vi "Subpanel - Helper.vi"() -> ()   [LabVIEW 2016]
uses:
  <vilib>/Utility/error.llb/DialogType.ctl
  <vilib>/SLL Toolkit/SLL Queued State Machine/Queue Driver/Create Queue.vi
  <vilib>/SLL Toolkit/SLL Queued State Machine/Queue Driver/Enqueue an Item to Queue.vi
  <vilib>/SLL Toolkit/SLL Queued State Machine/Queue Driver/Dequeue Queue.vi
  <vilib>/SLL Toolkit/SLL Queued State Machine/Queue Driver/Enqueue N Items.vi
  <vilib>/SLL Toolkit/SLL Queued State Machine/Queue Driver/Flush Queue.vi
  <vilib>/SLL Toolkit/SLL Queued State Machine/Queue Driver/Release Queue.vi
  <vilib>/SLL Toolkit/SLL Queued State Machine/SLL QSM.lvlib
panel:
  in  "STOP":bool
  in  "VI to load":string(combo)="Latch boolean simulation"
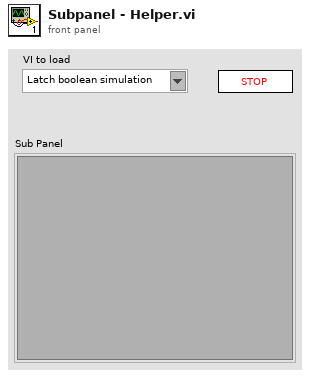
[diagram p1: front panel]
types:
  T1 = cluster{"Flags":cluster{"Source Code?":bool, "VI Inserted?":bool}, "VI Details":string[][], "VI Ref":refnum<vi>}
  T2 = typedef "DialogType.ctl" = u16
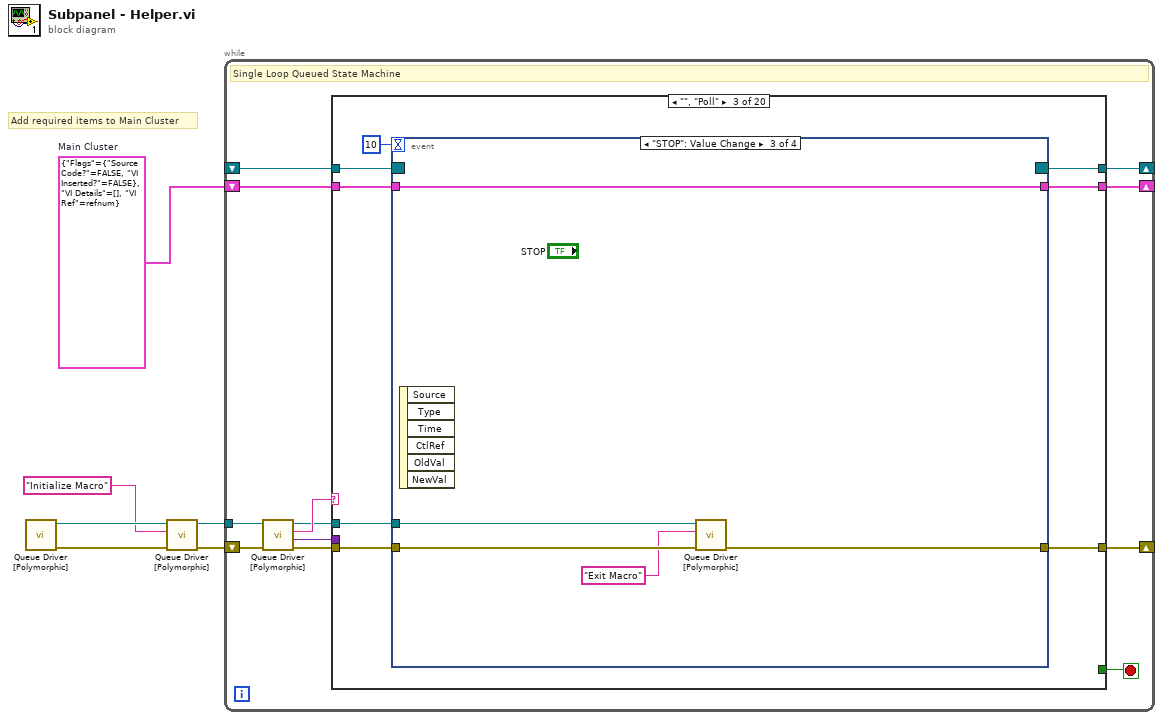
[diagram p0: block diagram]
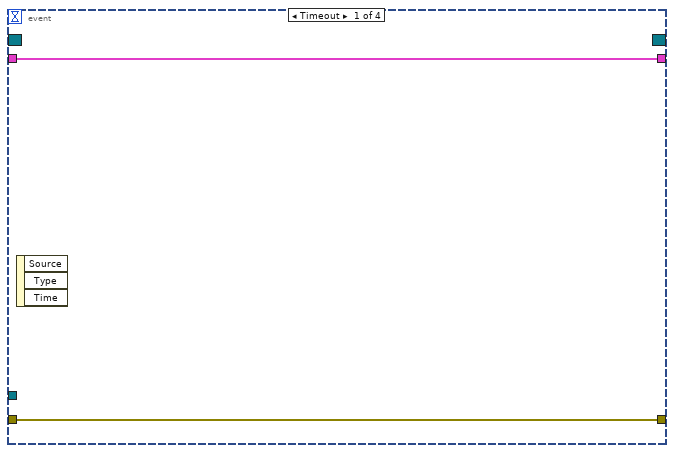
[diagram p4: hidden frame]
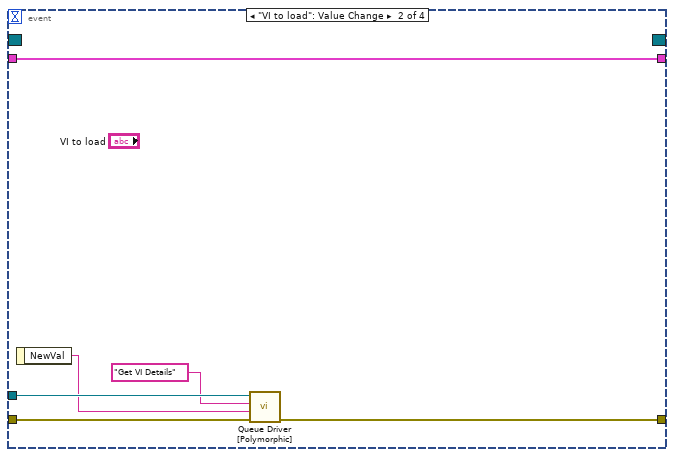
[diagram p5: hidden frame]
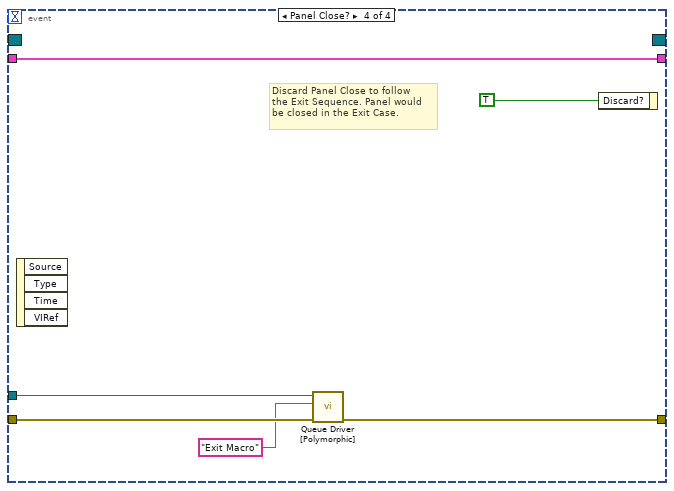
[diagram p6: hidden frame]
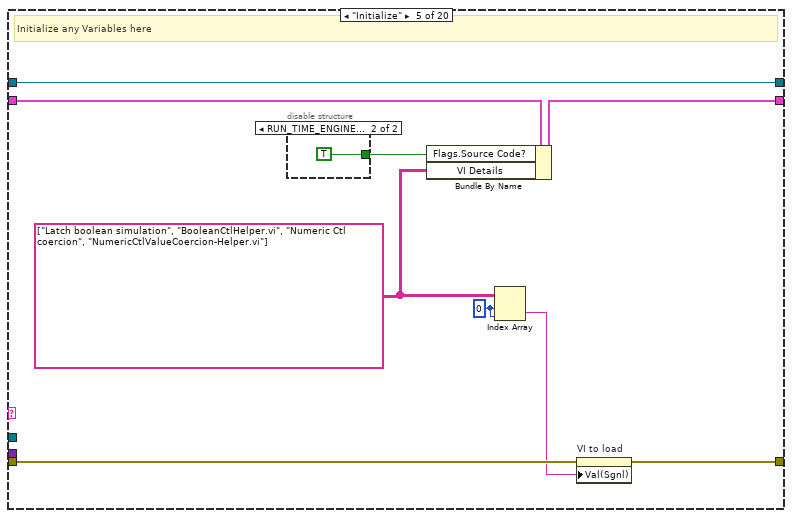
[diagram p8: hidden frame]
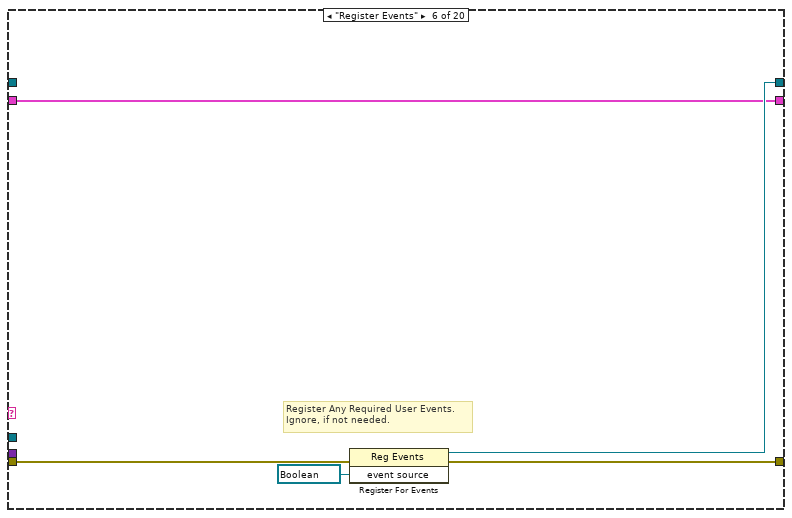
[diagram p10: hidden frame]
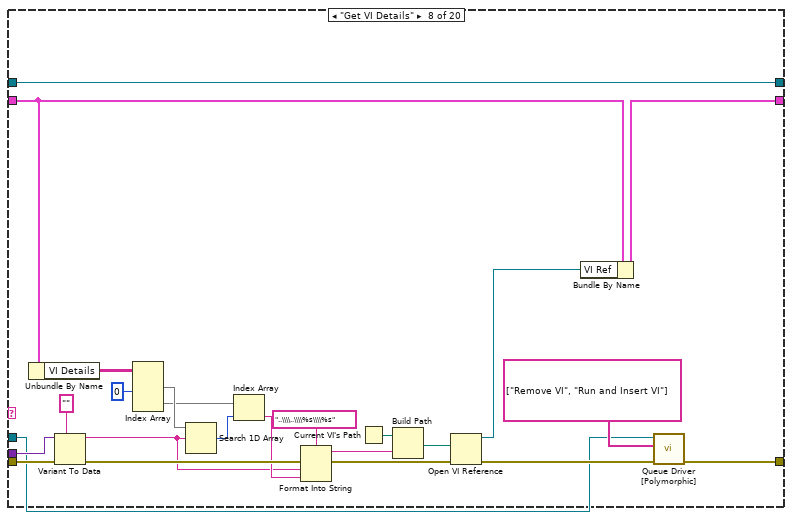
[diagram p12: hidden frame]
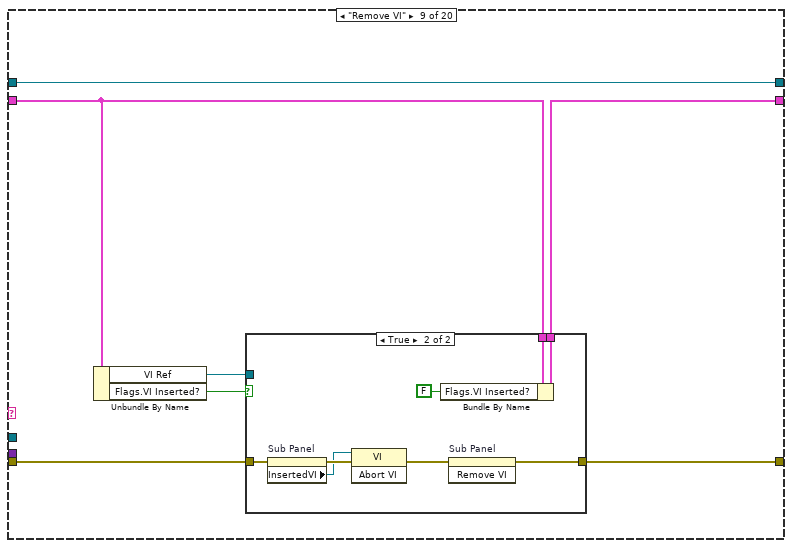
[diagram p13: hidden frame]
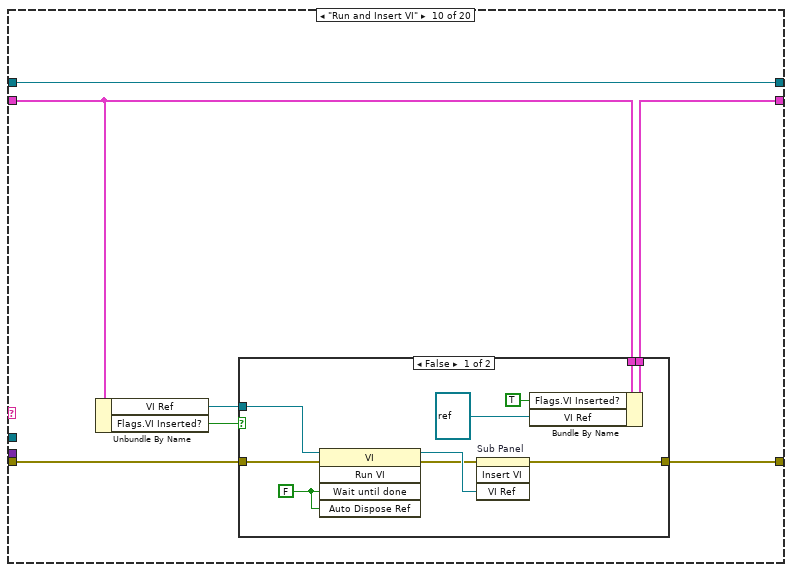
[diagram p15: hidden frame]
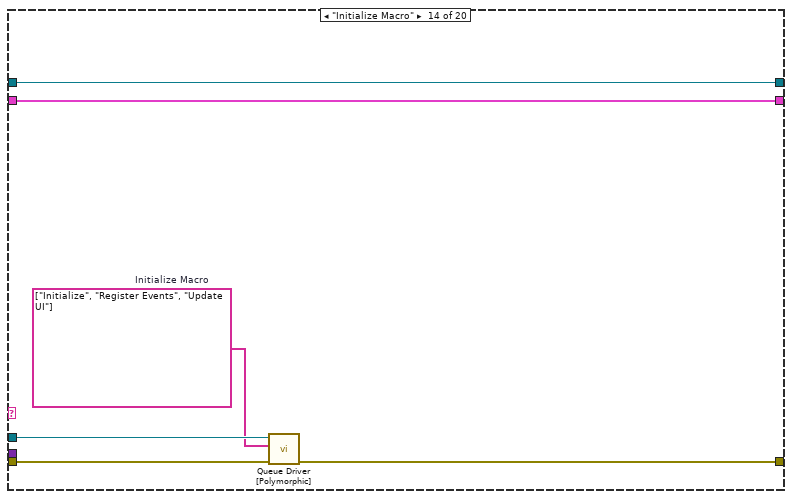
[diagram p20: hidden frame]
diagram:
  w3 = T1 {"Flags"={"Source Code?"=FALSE, "VI Inserted?"=FALSE}, "VI Details"=[], "VI Ref"=refnum}  # Main Cluster
  # "Add required items to Main Cluster"
  n1 = call-poly <vilib>:"Queue Driver [Polymorphic].vi"() -> ("Error Out"=w1:errorcluster, "Queue Ref"=w5:refnum<queue>)  [unwired: 10 in]
  n2 = call-poly <vilib>:"Queue Driver [Polymorphic].vi"("Error In"=w1, "Item to Add"="Initialize Macro", "Queue Ref In"=w5) -> ("Error Out"=w2:errorcluster, "Queue Ref Out"=w6:refnum<queue>)  [unwired: 7 in]
  n3 = while "SLL Queued State Machine" {
    shift-right: [w16] -> _
    shift-left: w2 -> [w18]
    shift-right: [w14] -> _
    shift-left: _ -> [w13]
    shift-right: [w12] -> _
    shift-left: w3 -> [w11]
    tunnel: w6 -> [w9]
    stop <- w15 stop-if-true
    # "Single Loop Queued State Machine"
    n4 = call-poly <vilib>:"Queue Driver [Polymorphic].vi"("Error In"=w18, "Queue Ref In"=w9) -> ("Error Out"=w17:errorcluster, "Data"=w7:variant, "Dequeue"=w10:string, "Queue Ref Out"=w8:refnum<queue>)  [unwired: 6 in]
    n5 = case "QSM Case Structure" shown="\"\", \"Poll\"" w10 {
      selector: w10 -> [_ _ _ _ _ _ _ _ _ _ _ _ _ _ _ _ w157 _ _ _]
      tunnel: w17 -> [w21 w24 w30 w54 w58 w69 w72 w96 w102 w120 w135 w138 w141 w145 w151 w156 w160 w172 w175 w188]
      tunnel: [w21 w24 w31 w54 w59 w68 w72 w77 w101 w117 w135 w138 w141 w144 w150 w156 w163 w170 w175 w184] -> w16
      tunnel: [_ _ _ _ _ _ _ _ _ _ _ _ _ _ _ _ _ _ _ TRUE] -> w15
      tunnel: [w20 w23 w29 w53 w63 w67 w71 w95 w103 w119 w134 w137 w140 w147 w153 w155 w166 w169 w174 w187] -> w14
      tunnel: w13 -> [w20 w23 w28 w53 w63 _ w71 w95 w103 w119 w134 w137 w140 w147 w153 w155 w166 w169 w174 w187]
      tunnel: [w19 w22 w26 w52 w60 w66 w70 w75 w97 w115 w133 w136 w139 w146 w152 w154 w165 w168 w173 w186] -> w12
      tunnel: w11 -> [w19 w22 w27 w52 w61 w66 w70 w76 w98 w116 w133 w136 w139 w146 w152 w154 w165 w168 w173 w186]
      tunnel: w8 -> [_ _ w25 _ _ _ _ w73 _ _ _ _ _ w143 w148 _ _ _ _ w177]
      tunnel: w7 -> [_ _ _ _ _ _ _ w93 _ _ _ _ _ _ _ _ _ _ _ _]
      frame "/--------------- Read Me -----------------/" {
        # "General Purpose Queue Based State Machine for Any Use Case (main application, module, pop up message etc)\n\nAdvantages:\n1. Lean Project Code Base (dependencies are in vilib).\n2. This template can be safely used in multiple parallel running modules without any issues.\n3. This template can also be safely used even in cases where the VI is configured to be a clone, where multiple \ninstances of the VI could be executing concurrently.\n\nHow to Use:\n1. Add necessary items to the Main Cluster.\n2. Use the Polymorphic Queue Driver for doing any queue operations. \n3. Add any required user events in the \"Register Events\" case. Ignore if not needed.\n4. Use \"Macros\" section for defining any list of state calls, which could be used in multiple places. \nEx: Initialize Macro, might be needed if we need to any reinitialization."
      }
      frame "/------------------ Poll -------------------/" {
      }
      frame "", "Poll" {
        n6 = event shown="[2] \"STOP\": Value Change" {
          selector: w28 -> [_ _ _ _]
          dyn-events: [_ _ _ _] -> w29
          timeout: 10 -> [_ _ _ _]
          tunnel: [w34 w37 w44 w50] -> w31
          tunnel: w30 -> [w34 w38 w45 w51]
          tunnel: w27 -> [w33 w40 w43 w49]
          tunnel: [w33 w40 w43 w49] -> w26
          tunnel: w25 -> [_ w39 w42 w47]
          event Timeout {
            n7 = event-data() -> ()  [unwired: 1 in, 3 out]
          }
          event "VI to load": Value Change {
            n8 = event-data() -> ("NewVal"=w35:string)  [unwired: 1 in]
            n9 = call-poly <vilib>:"Queue Driver [Polymorphic].vi"("Error In"=w38, "Data (Optional)"=w35, "Item to Add"="Get VI Details", "Queue Ref In"=w39) -> ("Error Out"=w37:errorcluster)  [unwired: 6 in, 1 out]
          }
          event "STOP": Value Change {
            n10 = event-data() -> ()  [unwired: 1 in, 6 out]
            n11 = call-poly <vilib>:"Queue Driver [Polymorphic].vi"("Error In"=w45, "Item to Add"="Exit Macro" ("Enqueue"), "Queue Ref In"=w42) -> ("Error Out"=w44:errorcluster)  [unwired: 7 in, 1 out]
          }
          event Panel Close? {
            # "Discard Panel Close to follow\nthe Exit Sequence. Panel would\nbe closed in the Exit Case."
            n12 = event-data() -> ()  [unwired: 1 in, 4 out]
            n13 = call-poly <vilib>:"Queue Driver [Polymorphic].vi"("Error In"=w51, "Item to Add"="Exit Macro" ("Enqueue"), "Queue Ref In"=w47) -> ("Error Out"=w50:errorcluster)  [unwired: 7 in, 1 out]
            n14 = event-data("Discard?"=TRUE) -> ()  [unwired: 1 in, 1 out]
          }
        }
      }
      frame "/--------------- Initialize -----------------/" {
      }
      frame "Initialize" {
        w56 = 0 ("index (row)")
        w57 = string[][] [["Latch boolean simulation", "BooleanCtlHelper.vi"], ["Numeric Ctl coercion", "NumericCtlValueCoercion-Helper.vi"]]
        # "Initialize any Variables here"
        n15 = disable-structure shown="RUN_TIME_ENGINE==False" {
          disable-tunnel: [_ TRUE] -> w62
          frame condition #0 {
          }
          frame condition #1 (active) {
          }
        }
        n16 = Bundle By Name(cluster=w61, "Flags.Source Code?"=w62, "VI Details"=w57) -> (w60:T1)
        n17 = Index Array(array=w57, index (row)=w56, index (col)=w56) -> (element=w55:string)
        n18 = property on="VI to load" class="CmbBox"(error in=w58, "Val(Sgnl)"=w55) -> (error out=w59:errorcluster)  [unwired: 1 in, 1 out]
      }
      frame "Register Events" {
        # "Register Any Required User Events. \nIgnore, if not needed."
        n19 = register-events(error in=w69, refnum<vi> refnum ("event source")) -> (reference out=w67:refnum<event-registration>, error out=w68:errorcluster)  [unwired: 1 in]
      }
      frame "/---------- Custom Case Splitter ----------/" {
      }
      frame "Get VI Details" {
        n20 = Unbundle By Name(w76) -> ("VI Details"=w91:string[][])
        n21 = Variant To Data(error in=w96, type="", Variant=w93) -> (data=w81:string, error out=w85:errorcluster)
        n22 = Index Array(array=w91, index (col) #1=0 ("disabled index (col)")) -> (element #1=w89:string[], element #2=w88:string[])  [unwired: 3 in]
        n23 = Search 1D Array(1D array=w89, element=w81) -> (index of element=w87:i32)  [unwired: 1 in]
        n24 = Index Array(array=w88, index=w87) -> (element=w83:string)
        n25 = Format Into String(format string="..\\\\..\\\\%s\\\\%s", error in=w85, w81, w83) -> (resulting string=w80:string, error out=w84:errorcluster)  [unwired: 1 in]
        n26 = Current VI's Path() -> (path=w86:path)
        n27 = Build Path(base path=w86, name or relative path=w80) -> (appended path=w79:path)
        n28 = Open VI Reference(vi path=w79, error in (no error)=w84) -> (vi reference=w74:refnum<vi>, error out=w78:errorcluster)  [unwired: 4 in]
        n29 = Bundle By Name(cluster=w76, "VI Ref"=w74) -> (w75:T1)
        n30 = call-poly <vilib>:"Queue Driver [Polymorphic].vi"("Error In"=w78, "Enqueue N"=string[] ["Remove VI", "Run and Insert VI"], "Queue Ref In"=w73) -> ("Error Out"=w77:errorcluster)  [unwired: 7 in, 1 out]
      }
      frame "Remove VI" {
        n31 = Unbundle By Name(w98) -> ("VI Ref"=w99:refnum<vi>, "Flags.VI Inserted?"=w100:bool)
        n32 = case shown="True" w100 {
          tunnel: w102 -> [w105 w113]
          tunnel: [w105 w109] -> w101
          tunnel: w99 -> [_ _]
          tunnel: w98 -> [w104 w108]
          tunnel: [w104 w107] -> w97
          frame False {
          }
          frame True {
            n33 = property on="Sub Panel" class="SubPnl"(error in=w113) -> (error out=w112:errorcluster, "InsertedVI"=w111:refnum<vi>)  [unwired: 1 in, 1 out]
            n34 = invoke class="VI" method="Abort VI"(reference=w111, error in=w112) -> (error out=w110:errorcluster)  [unwired: 1 in, 2 out]
            n35 = Bundle By Name(cluster=w108, "Flags.VI Inserted?"=FALSE) -> (w107:T1)
            n36 = invoke on="Sub Panel" class="SubPnl" method="Remove VI"(error in=w110) -> (error out=w109:errorcluster)  [unwired: 2 in, 2 out]
          }
        }
      }
      frame "Run and Insert VI" {
        n37 = Unbundle By Name(w116) -> ("VI Ref"=w118:refnum<vi>, "Flags.VI Inserted?"=w114:bool)
        n38 = case shown="False" w114 {
          tunnel: w120 -> [w130 w131]
          tunnel: w118 -> [w129 _]
          tunnel: [w126 w131] -> w117
          tunnel: w116 -> [w123 w132]
          tunnel: [w122 w132] -> w115
          frame False {
            w125 = FALSE ("Wait Until Done")
            n39 = invoke class="VI" method="Run VI"(reference=w129, error in=w130, "Wait until done"=w125, "Auto Dispose Ref"=w125) -> (reference out=w128:refnum<vi>, error out=w127:errorcluster)  [unwired: 1 in, 3 out]
            n40 = invoke on="Sub Panel" class="SubPnl" method="Insert VI"(error in=w127, "VI Ref"=w128) -> (error out=w126:errorcluster)  [unwired: 2 in, 3 out]
            n41 = Bundle By Name(cluster=w123, "Flags.VI Inserted?"=TRUE, "VI Ref"=refnum<vi> refnum) -> (w122:T1)
          }
          frame True {
          }
        }
      }
      frame "/-------------- User Interface --------------/" {
        # "Duplicate this case to create additional case splitters for readability"
      }
      frame "Update UI" {
        # "Update Front Panel Controls in this Case"
      }
      frame "/----------------- Macros -----------------/" {
      }
      frame "Initialize Macro" {
        w142 = string[] ["Initialize", "Register Events", "Update UI"]  # Initialize Macro
        n42 = call-poly <vilib>:"Queue Driver [Polymorphic].vi"("Error In"=w145, "Enqueue N"=w142, "Queue Ref In"=w143) -> ("Error Out"=w144:errorcluster)  [unwired: 7 in, 1 out]
      }
      frame "Exit Macro" {
        n43 = call-poly <vilib>:"Queue Driver [Polymorphic].vi"("Error In"=w151, "Enqueue N"=string[] ["Remove VI", "Exit"], "Queue Ref In"=w148) -> ("Error Out"=w150:errorcluster)  [unwired: 7 in, 1 out]
      }
      frame "/-------------- Error Handler--------------/" {
      }
      frame Default {
        # "Undefined Case/Spelling Errors - Show Message to Developer"
        n44 = property class="VI"(error in=w160) -> (error out=w159:errorcluster, "Name"=w158:string)  [unwired: 1 in, 1 out]
        n45 = Format Into String(format string="\"%s\" in the VI - %s" ("message"), initial string="Undefined case - ", error in=w159, w157, w158) -> (resulting string=w161:string, error out=w163:errorcluster)
        n46 = One Button Dialog(message=w161) -> ()  [unwired: 1 in, 1 out]
      }
      frame "Error" {
        w167 = T2 2 items=["no dialog", "OK message", "continue or stop message", "OK message + warnings", "continue/stop + warnings"] ("type of dialog (OK msg:1)")
        # "Handle the Error"
        n47 = call <vilib>:"Simple Error Handler.vi"("type of dialog (OK msg:1)"=w167, "error in (no error)"=w172) -> ("error out"=w171:errorcluster)  [unwired: 3 in, 4 out]
        n48 = call <vilib>:"Clear Errors.vi"("error in (no error)"=w171) -> ("error out"=w170:errorcluster)  [unwired: 5 in, 1 out]
      }
      frame "/------------------- Exit --------------------/" {
      }
      frame "Exit" {
        n49 = call-poly <vilib>:"Queue Driver [Polymorphic].vi"("Error In"=w188, "Queue Ref In"=w177) -> ("Error Out"=w189:errorcluster, "Queue Ref Out"=w176:refnum<queue>)  [unwired: 7 in, 1 out]
        n50 = Unbundle By Name(w186) -> ("Flags.Source Code?"=w179:bool)
        n51 = call-poly <vilib>:"Queue Driver [Polymorphic].vi"("Error In"=w189, "Queue Ref In"=w176) -> ("Error Out"=w185:errorcluster)  [unwired: 9 in]
        n52 = Call Chain() -> (call chain=w183:string[])
        n53 = Array Size(array=w183) -> (size(s)=w182:i32)
        n54 = Equal?(x=w182, y=1) -> (x = y?=w180:bool)
        n55 = And(x=w179, y=w180) -> (x .and. y?=w178:bool)
        n56 = case "Skip Panel Close when in Source\nCode and is the top most caller" shown="False" w178 {
          tunnel: w185 -> [w192 w194]
          tunnel: [w193 w194] -> w184
          frame False {
            # "Close Panel"
            n57 = invoke class="VI" method="FP.Close"() -> (error out=w191:errorcluster)  [unwired: 3 in, 2 out]
            n58 = Merge Errors(w192, w191) -> (w193:errorcluster)
          }
          frame True {
            # "Do Not Close Panel"
          }
        }
      }
    }
  }
